vi "Unified Actor And Unified Msgs.vi"(6 "Current Persistent Unified Msgs":T1, 9 "Current Persistent Unified Actor":refnum<class "Actor.lvclass">, 10 "Decorator Actors":refnum<class "Actor.lvclass">[](array[class])) -> (1 "Unified Msgs":T1, 2 "Unified Actor":refnum<class "Actor.lvclass">)   [LabVIEW 2025, in "jettl.lvlib"]
uses:
  jettl.lvlib
  Actor/Actor.lvclass
  Msgs.ctl
  Msg/Msg.lvclass
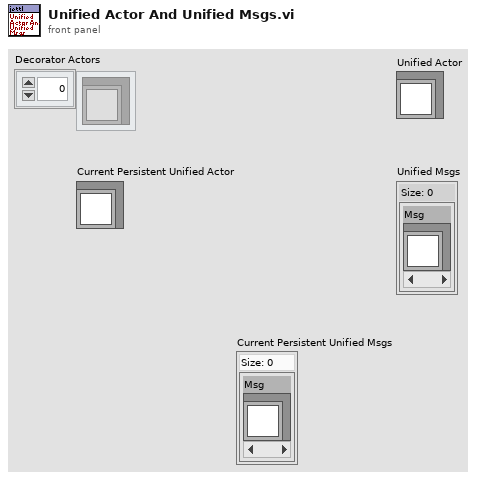
[diagram p1: front panel]
types:
  T1 = typedef "jettl.lvlib/Msgs.ctl" = set{refnum<class "Msg.lvclass">}
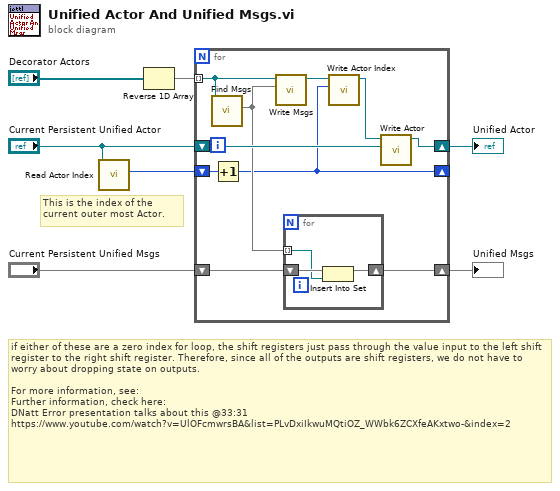
[diagram p0: block diagram]
diagram:
  # "if either of these are a zero index for loop, the shift registers just pass through the value input to the left shift register to the right shift register. Therefore, since all of the outputs are shift registers, we do not have to worry about dropping state on outputs.\n\nFor more information, see:\nFurther information, check here:\nDNatt Error presentation talks about this @33:31\nhttps://www.youtube.com/watch?v=UlOFcmwrsBA&list=PLvDxiIkwuMQtiOZ_WWbk6ZCXfeAKxtwo-&index=2"
  # "This is the index of the current outer most Actor."
  n1 = call-dynamic "Read Actor Index.vi"("Actor in"="Current Persistent Unified Actor") -> ("Actor Index"=w1:i32)  [unwired: 10 in]
  n2 = Reverse 1D Array(array="Decorator Actors") -> (reversed array=w7:refnum<class "Actor.lvclass">[])
  n3 = for {
    tunnel: w7 -> [w15] mode=indexing
    shift-right: [w16] -> w4
    shift-left: "Current Persistent Unified Actor" -> [w17]
    shift-right: [w13] -> w3
    shift-left: "Current Persistent Unified Msgs" -> [w14]
    shift-right: [w8] -> _
    shift-left: w1 -> [w9]
    n4 = call-dynamic "Find Msgs.vi"("Actor in"=w15) -> ("Msgs"=w12:T1)  [unwired: 10 in]
    n5 = Increment(x=w9) -> (x+1=w8:i32)
    n6 = call-dynamic "Write Msgs.vi"("Msgs"=w12, "Actor in"=w15) -> ("Actor out"=w11:refnum<class "Actor.lvclass">)  [unwired: 9 in]
    n7 = for {
      shift-right: [w19] -> w13
      shift-left: w14 -> [w20]
      tunnel: w12 -> [w18] mode=indexing
      n8 = Insert Into Set(10:w18, 11:w20) -> (3:w19:T1)  [unwired: 1 out]
    }
    n9 = call-dynamic "Write Actor Index.vi"("Actor Index"=w8, "Actor in"=w11) -> ("Actor out"=w10:refnum<class "Actor.lvclass">)  [unwired: 9 in]
    n10 = call-dynamic "Write Actor.vi"("Actor"=w17, "Actor in"=w10) -> ("Actor out"=w16:refnum<class "Actor.lvclass">)  [unwired: 9 in]
  }
  "Unified Actor" <- w4
  "Unified Msgs" <- w3
